vi "stage_setposition_wait.vi"(8 "error in (no error)":errorcluster, 9 "speeds":T1={"speedx"=4.0, "speedy"=4.0, "speedz"=4.0} {"speedx" min=0 max=4; "speedy" min=0 max=4; "speedz" min=0 max=4}, 10 "Position in[µm]":T2, 11 "Stage reference in":T3) -> (0 "error out":errorcluster, 3 "Stage reference out":T3)   [LabVIEW 2018]
uses:
  stage_reference_type.ctl
  <userlib>/stepper/velocity settings.ctl
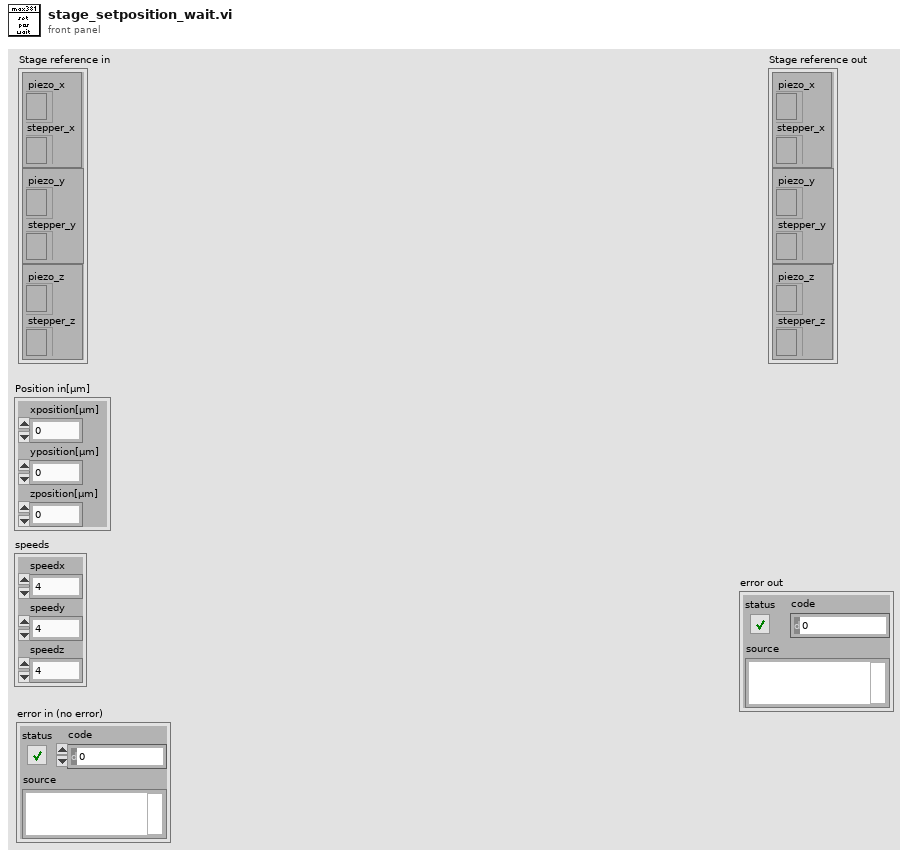
[diagram p1: front panel]
types:
  T1 = cluster{"speedx":sgl, "speedy":sgl, "speedz":sgl}
  T2 = cluster{"xposition[µm]":sgl, "yposition[µm]":sgl, "zposition[µm]":sgl}
  T3 = typedef "stage_reference_type.ctl" = cluster{cluster{"piezo_x":refnum<k7>, "stepper_x":refnum<k7>}, cluster{"piezo_y":refnum<k7>, "stepper_y":refnum<k7>}, cluster{"piezo_z":refnum<k7>, "stepper_z":refnum<k7>}}
  T4 = typedef "velocity settings.ctl" = cluster{"pfMinVel":sgl, "pfAccn":sgl, "pfMaxVel":sgl}
  T5 = cluster{"piezo_x":refnum<k7>, "stepper_x":refnum<k7>}
  T6 = cluster{"piezo_y":refnum<k7>, "stepper_y":refnum<k7>}
  T7 = cluster{"piezo_z":refnum<k7>, "stepper_z":refnum<k7>}
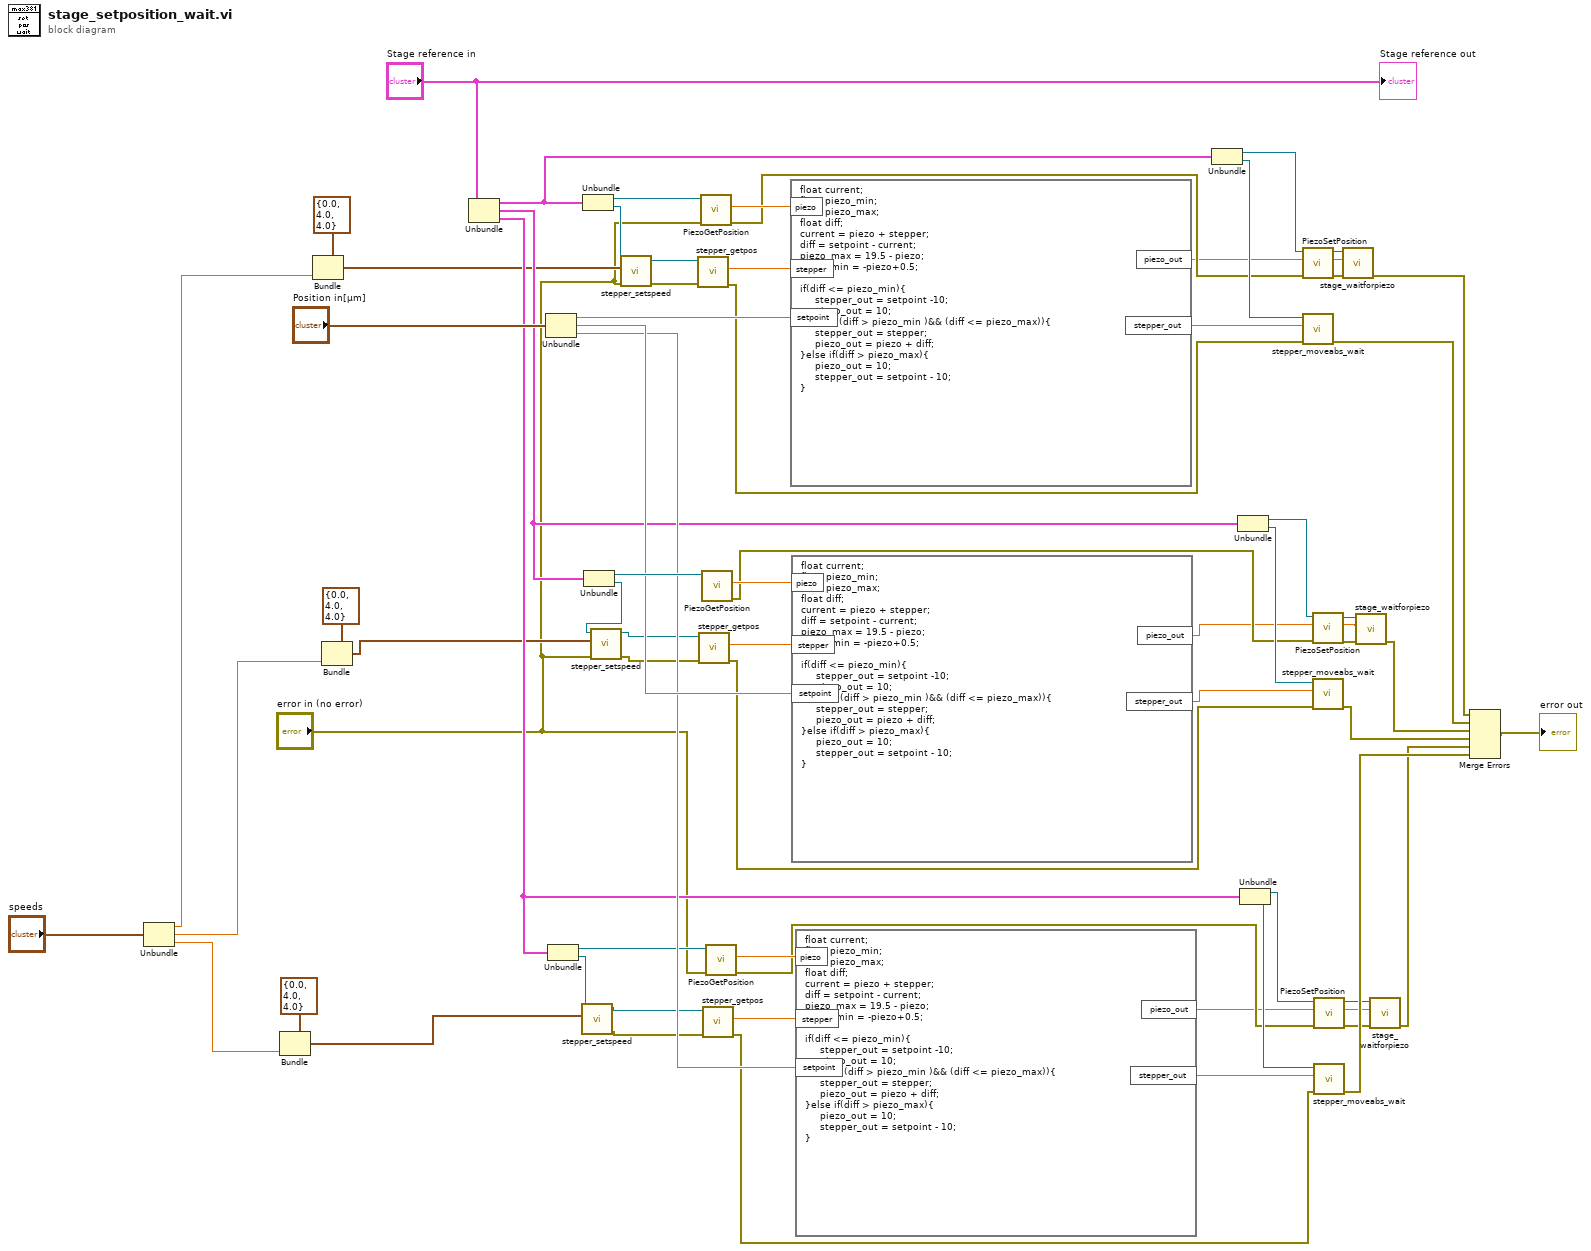
[diagram p0: block diagram]
diagram:
  n1 = Unbundle("speeds") -> ("speedx"=w7:sgl, "speedy"=w18:sgl, "speedz"=w6:sgl)
  n2 = Bundle(cluster=T4 {"pfMinVel"=0.0, "pfAccn"=4.0, "pfMaxVel"=4.0} ("velocity parameters in"), "pfMaxVel"=w6) -> (w9:T4)  [unwired: 2 in]
  n3 = Bundle(cluster=T4 {"pfMinVel"=0.0, "pfAccn"=4.0, "pfMaxVel"=4.0} ("velocity parameters in"), "pfMaxVel"=w7) -> (w17:T4)  [unwired: 2 in]
  n4 = Bundle(cluster=T4 {"pfMinVel"=0.0, "pfAccn"=4.0, "pfMaxVel"=4.0} ("velocity parameters in"), "pfMaxVel"=w18) -> (w8:T4)  [unwired: 2 in]
  n5 = Unbundle("Stage reference in") -> (w50:T5, w51:T6, w52:T7)
  n6 = Unbundle("Position in[µm]") -> ("xposition[µm]"=w62:sgl, "yposition[µm]"=w55:sgl, "zposition[µm]"=w54:sgl)
  n7 = Unbundle(w52) -> ("piezo_z"=w53:refnum<k7>, "stepper_z"=w12:refnum<k7>)
  n8 = call <userlib>:"stepper_setspeed.vi"("velocity parameters in"=w9, "reference"=w12) -> ("error out"=w10:errorcluster, "reference out"=w11:refnum<k7>)  [unwired: 7 in, 1 out]
  n9 = Unbundle(w50) -> ("piezo_x"=w66:refnum<k7>, "stepper_x"=w65:refnum<k7>)
  n10 = Unbundle(w51) -> ("piezo_y"=w61:refnum<k7>, "stepper_y"=w5:refnum<k7>)
  n11 = call <userlib>:"stepper_setspeed.vi"("error in (no error)"="error in (no error)", "velocity parameters in"=w8, "reference"=w5) -> ("error out"=w3:errorcluster, "reference out"=w4:refnum<k7>)  [unwired: 6 in, 1 out]
  n12 = call <userlib>:"stepper_setspeed.vi"("error in (no error)"="error in (no error)", "velocity parameters in"=w17) -> ("error out"=w2:errorcluster)  [unwired: 7 in, 2 out]
  n13 = call <userlib>:"stepper_getpos.vi"("error in (no error)"=w2, "reference"=w65) -> ("error out"=w39:errorcluster, "pfPosition[µm]"=w63:sgl)  [unwired: 7 in, 1 out]
  n14 = call <userlib>:"stepper_getpos.vi"("error in (no error)"=w3, "reference"=w4) -> ("error out"=w36:errorcluster, "pfPosition[µm]"=w59:sgl)  [unwired: 7 in, 1 out]
  n15 = call <userlib>:"PiezoGetPosition.vi"("error in (no error)"="error in (no error)", "reference"=w66) -> ("error out"=w40:errorcluster, "Position"=w64:sgl)  [unwired: 3 in, 1 out]
  n16 = call <userlib>:"PiezoGetPosition.vi"("reference"=w61) -> ("error out"=w37:errorcluster, "Position"=w60:sgl)  [unwired: 4 in, 1 out]
  n17 = call <userlib>:"stepper_getpos.vi"("error in (no error)"=w10, "reference"=w11) -> ("error out"=w33:errorcluster, "pfPosition[µm]"=w57:sgl)  [unwired: 7 in, 1 out]
  n18 = call <userlib>:"PiezoGetPosition.vi"("error in (no error)"="error in (no error)", "reference"=w53) -> ("error out"=w34:errorcluster, "Position"=w58:sgl)  [unwired: 3 in, 1 out]
  n19 = formula code="float current;\nfloat piezo_min;\nfloat piezo_max;\nfloat diff;\ncurrent = piezo + stepper;\ndiff = setpoint - current;\npiezo_max = 19.5 - piezo;\npiezo_min = -piezo+0.5;\n\nif(diff <= piezo_min){\n     stepper_out = setpoint -10;\n     piezo_out = 10;\n}else if((diff > piezo_min )&& (diff <= piezo_max)){\n     stepper_out = stepper;\n     piezo_out = piezo + diff;\n}else if(diff > piezo_max){\n     piezo_out = 10;\n     stepper_out = setpoint - 10;\n}"("piezo"=w64, "stepper"=w63, "setpoint"=w62) -> ("piezo_out"=w22:dbl, "stepper_out"=w48:dbl)
  n20 = formula code="float current;\nfloat piezo_min;\nfloat piezo_max;\nfloat diff;\ncurrent = piezo + stepper;\ndiff = setpoint - current;\npiezo_max = 19.5 - piezo;\npiezo_min = -piezo+0.5;\n\nif(diff <= piezo_min){\n     stepper_out = setpoint -10;\n     piezo_out = 10;\n}else if((diff > piezo_min )&& (diff <= piezo_max)){\n     stepper_out = stepper;\n     piezo_out = piezo + diff;\n}else if(diff > piezo_max){\n     piezo_out = 10;\n     stepper_out = setpoint - 10;\n}"("piezo"=w60, "stepper"=w59, "setpoint"=w55) -> ("piezo_out"=w25:dbl, "stepper_out"=w41:dbl)
  n21 = formula code="float current;\nfloat piezo_min;\nfloat piezo_max;\nfloat diff;\ncurrent = piezo + stepper;\ndiff = setpoint - current;\npiezo_max = 19.5 - piezo;\npiezo_min = -piezo+0.5;\n\nif(diff <= piezo_min){\n     stepper_out = setpoint -10;\n     piezo_out = 10;\n}else if((diff > piezo_min )&& (diff <= piezo_max)){\n     stepper_out = stepper;\n     piezo_out = piezo + diff;\n}else if(diff > piezo_max){\n     piezo_out = 10;\n     stepper_out = setpoint - 10;\n}"("piezo"=w58, "stepper"=w57, "setpoint"=w54) -> ("piezo_out"=w29:dbl, "stepper_out"=w46:dbl)
  n22 = Unbundle(w50) -> ("piezo_x"=w49:refnum<k7>, "stepper_x"=w47:refnum<k7>)
  n23 = Unbundle(w51) -> ("piezo_y"=w42:refnum<k7>, "stepper_y"=w43:refnum<k7>)
  n24 = Unbundle(w52) -> ("piezo_z"=w45:refnum<k7>, "stepper_z"=w44:refnum<k7>)
  n25 = call <userlib>:"PiezoSetPosition.vi"("error in (no error)"=w40, "pos in"=w22, "reference"=w49) -> ("error out"=w23:errorcluster, "reference out"=w21:refnum<k7>)  [unwired: 3 in]
  n26 = call <userlib>:"stepper_moveabs_wait.vi"("error in (no error)"=w39, "fAbsPos[µm]"=w48, "reference"=w47) -> ("error out"=w38:errorcluster)  [unwired: 7 in, 1 out]
  n27 = call <userlib>:"PiezoSetPosition.vi"("error in (no error)"=w37, "pos in"=w25, "reference"=w42) -> ("error out"=w27:errorcluster, "reference out"=w24:refnum<k7>)  [unwired: 3 in]
  n28 = call <userlib>:"stepper_moveabs_wait.vi"("error in (no error)"=w36, "fAbsPos[µm]"=w41, "reference"=w43) -> ("error out"=w35:errorcluster)  [unwired: 7 in, 1 out]
  n29 = call <userlib>:"PiezoSetPosition.vi"("error in (no error)"=w34, "pos in"=w29, "reference"=w45) -> ("error out"=w30:errorcluster, "reference out"=w28:refnum<k7>)  [unwired: 3 in]
  n30 = call <userlib>:"stepper_moveabs_wait.vi"("error in (no error)"=w33, "fAbsPos[µm]"=w46, "reference"=w44) -> ("error out"=w32:errorcluster)  [unwired: 7 in, 1 out]
  n31 = call "stage_waitforpiezo.vi"("error in (no error)"=w23, "Position"=w22, "reference"=w21) -> ("error out"=w20:errorcluster)  [unwired: 7 in, 1 out]
  n32 = call "stage_waitforpiezo.vi"("error in (no error)"=w27, "Position"=w25, "reference"=w24) -> ("error out"=w26:errorcluster)  [unwired: 7 in, 1 out]
  n33 = call "stage_waitforpiezo.vi"("error in (no error)"=w30, "Position"=w29, "reference"=w28) -> ("error out"=w19:errorcluster)  [unwired: 7 in, 1 out]
  n34 = Merge Errors(w20, w38, w26, w35, w19, w32) -> (→"error out":errorcluster)
  "Stage reference out" <- "Stage reference in"
